vi "Add IL Action.vi"(5 "Insert infront (F)":bool, 8 "error in (no error)":errorcluster, 10 "IL Action in":refnum<class "IL Action.lvclass">, 11 "Interlock in":refnum<class "Interlock.lvclass">) -> (0 "error out":errorcluster, 3 "Interlock out":refnum<class "Interlock.lvclass">)   [LabVIEW 2015, in "Interlocks.lvlib" / "Interlock.lvclass"]
uses:
  Interlock.lvclass
  IL Action/IL Action.lvclass
  Interlock.lvclass/Interlock.ctl
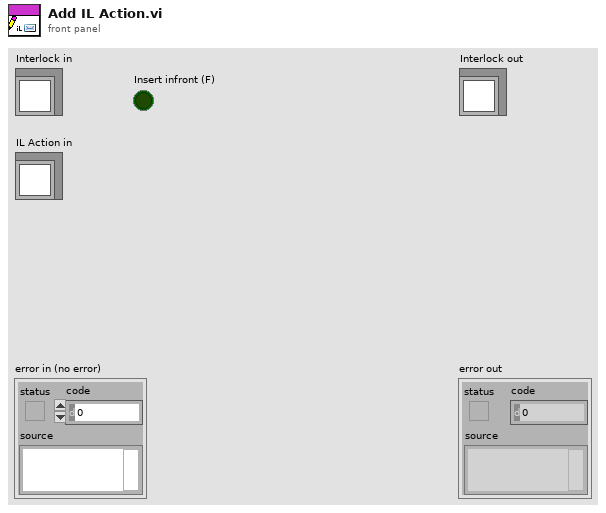
[diagram p1: front panel]
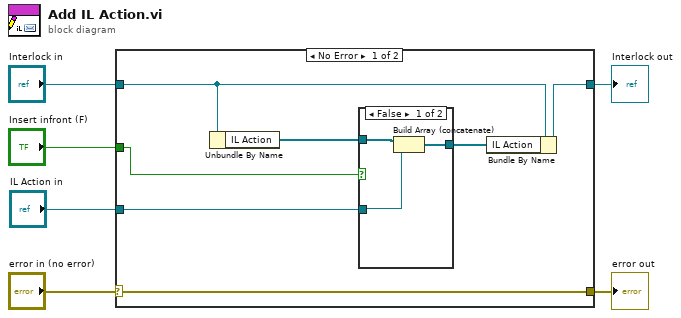
[diagram p0: block diagram]
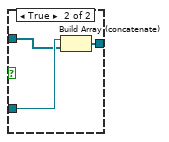
[diagram p2: hidden frame]
diagram:
  n1 = case shown="No Error" "error in (no error)" {
    selector: "error in (no error)" -> [w8 w20]
    tunnel: [w8 w20] -> w5
    tunnel: [w10 w21] -> w3
    tunnel: "Interlock in" -> [w13 w21]
    tunnel: "Insert infront (F)" -> [w9 _]
    tunnel: "IL Action in" -> [w7 _]
    frame No Error {
      n2 = Unbundle By Name(w13) -> ("IL Action"=w12:refnum<class "IL Action.lvclass">[])
      n3 = case shown="False" w9 {
        tunnel: w12 -> [w16 w18]
        tunnel: w7 -> [w14 w19]
        tunnel: [w15 w17] -> w11
        frame False {
          n4 = Build Array (concatenate)(w16, w14) -> (w15:refnum<class "IL Action.lvclass">[])
        }
        frame True {
          n5 = Build Array (concatenate)(w19, w18) -> (w17:refnum<class "IL Action.lvclass">[])
        }
      }
      n6 = Bundle By Name(cluster=w13, "IL Action"=w11) -> (w10:refnum<class "Interlock.lvclass">)
    }
    frame Error {
    }
  }
  "error out" <- w5
  "Interlock out" <- w3
